vi "Lab2.vi"() -> ()   [LabVIEW 2019]
uses:
  <vilib>/Instr/_visa.llb/VISA Configure Serial Port (Instr).vi
  <vilib>/Utility/file.llb/Write Delimited Spreadsheet (DBL).vi
panel:
  out "Background":bool
  out "Delta":bool
  out "Nominal":bool
  out "UV Index":dbl
  out "array w/ subset deleted":dbl[][](array[numeric])
  out "Lux Index":dbl
  out "UV Chart":dbl(graph)
  out "Lux Chart":dbl(graph)
  in  "?":bool
  in  "Arduino COM Port":refnum<visa-resource-name>="COM3"
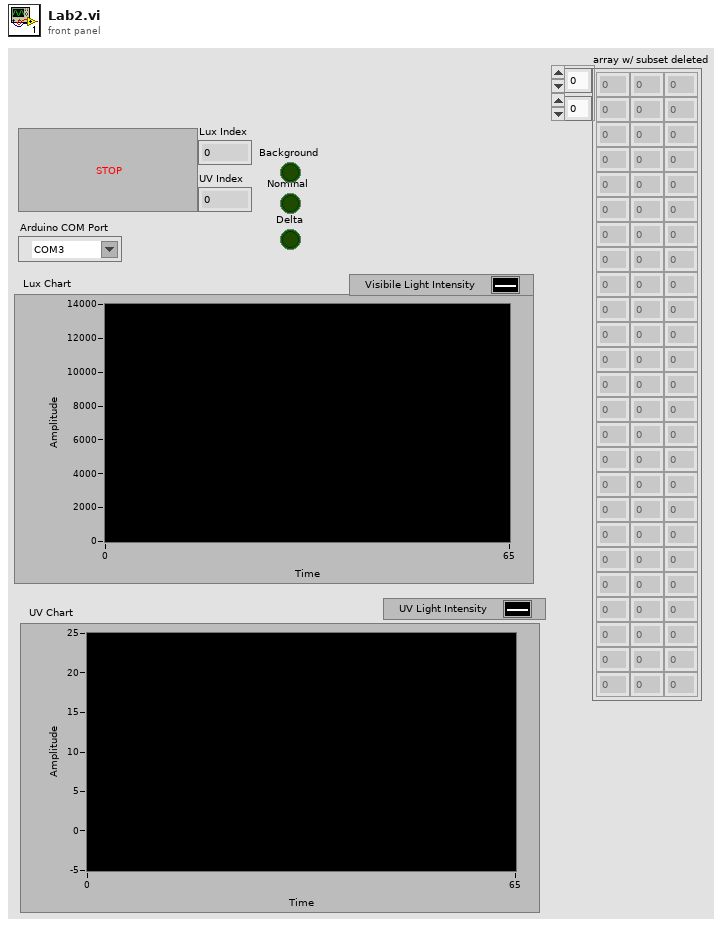
[diagram p1: front panel]
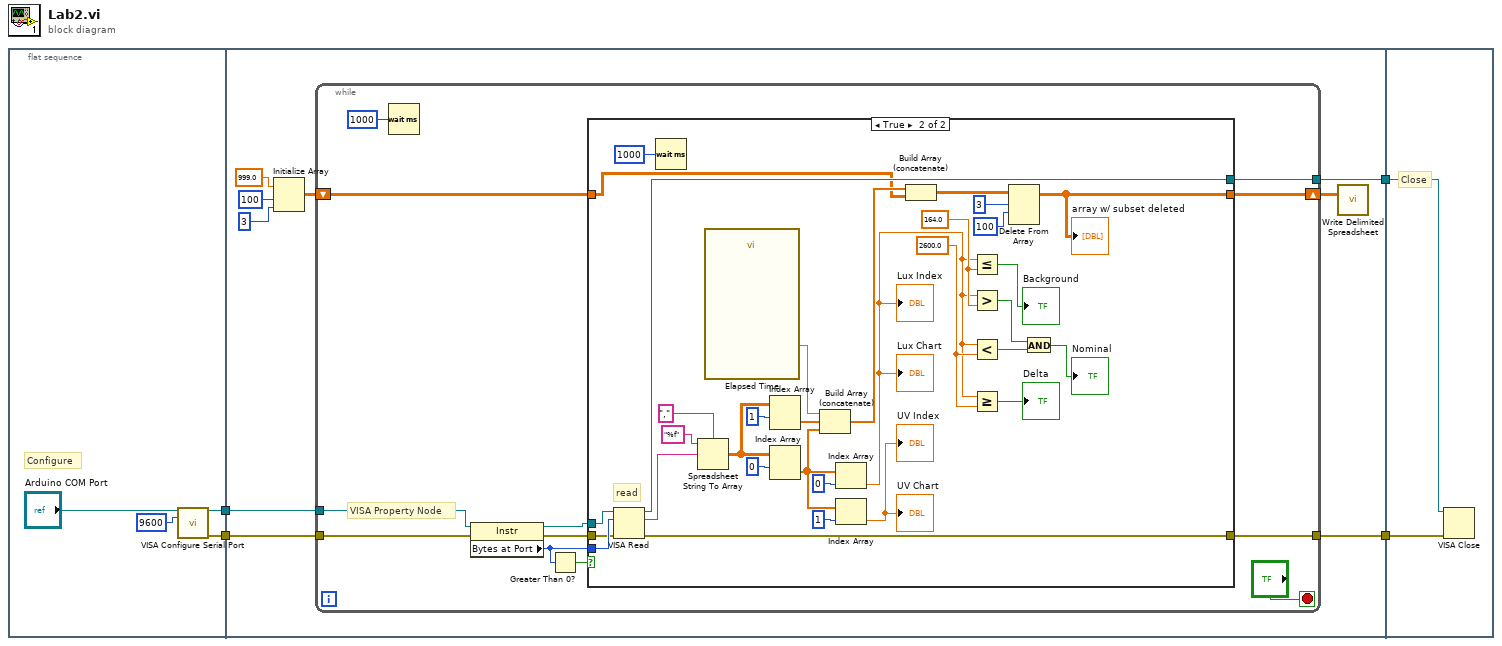
[diagram p0: block diagram]
diagram:
  n1 = flat-sequence {
    tunnel: [w6] -> w4
    tunnel: [w5] -> w3
    tunnel: w4 -> [w17]
    tunnel: [w16] -> w2
    tunnel: w3 -> [w15]
    tunnel: [w14] -> w1
    tunnel: w2 -> [w66]
    tunnel: w1 -> [w65]
    frame #0 {
      # "Configure"
      n2 = call-poly "VISA Configure Serial Port"("VISA resource name"="Arduino COM Port", "baud rate (9600)"=u32 9600) -> ("VISA resource name out"=w6:refnum<visa-resource-name>, "error out"=w5:errorcluster)  [unwired: 12 in]
    }
    frame #1 {
      n3 = Initialize Array(999.0 ("element"), 100 ("dimension size"), 3 ("dimension size")) -> (w10:dbl[][])
      n4 = while {
        tunnel: w17 -> [w21]
        tunnel: [w24] -> w16
        tunnel: w15 -> [w20]
        tunnel: [w22] -> w14
        shift-right: [w18] -> w9
        shift-left: w10 -> [w19]
        stop <- "?" stop-if-true
        # "VISA Property Node"
        n5 = Wait (ms)(milliseconds to wait=u32 1000) -> ()  [unwired: 1 out]
        n6 = property class="Instr"(reference=w21, error in=w20) -> (reference out=w28:refnum<visa-resource-name>, error out=w23:errorcluster, "Bytes at Port"=w27:u32)
        n7 = Greater Than 0?(x=w27) -> (x > 0?=w29:bool)
        n8 = case shown="True" w29 {
          tunnel: w28 -> [w32 w64]
          tunnel: [w32 w63] -> w24
          tunnel: w27 -> [_ w59]
          tunnel: w23 -> [w31 w58]
          tunnel: [w31 w57] -> w22
          tunnel: w19 -> [w30 w50]
          tunnel: [w30 w46] -> w18
          frame False {
          }
          frame True {
            w34 = 2600.0 ("y")
            w39 = 164.0 ("y")
            # "read"
            n9 = VISA Read(VISA resource name=w64, byte count=w59, error in (no error)=w58) -> (VISA resource name out=w63:refnum<visa-resource-name>, read buffer=w62:string, error out=w57:errorcluster)  [unwired: 1 out]
            n10 = Wait (ms)(milliseconds to wait=u32 1000) -> ()  [unwired: 1 out]
            n11 = Spreadsheet String To Array(delimiter (Tab)=",", format string="%f", spreadsheet string=w62) -> (array=w45:dbl[][])  [unwired: 1 in]
            n12 = call "Elapsed Time"() -> ("Elapsed Time (s)"=w53:dbl)  [unwired: 12 in, 7 out]
            n13 = Index Array(array=w45, index (row)=1) -> (element=w52:dbl[])  [unwired: 1 in]
            n14 = Index Array(array=w45, index (row)=0) -> (element=w44:dbl[])  [unwired: 1 in]
            n15 = Build Array (concatenate)(w53, w52, w44) -> (w51:dbl[])
            n16 = Index Array(array=w44, index=0) -> (element=w33:dbl)
            "Lux Chart" <- w33
            "Lux Index" <- w33
            n17 = Index Array(array=w44, index=1) -> (element=→"UV Chart" →"UV Index":dbl)
            n18 = Build Array (concatenate)(w51, w50) -> (w49:dbl[][])
            n19 = Less Or Equal?(x=w33, y=w39) -> (x <= y?=→"Background":bool)
            n20 = Greater?(x=w33, y=w39) -> (0:w38:bool)
            n21 = Less?(x=w33, y=w34) -> (x < y?=w36:bool)
            n22 = Greater Or Equal?(x=w33, y=w34) -> (x >= y?=→"Delta":bool)
            n23 = Delete From Array(array=w49, length=3, index (row)=100) -> (array with subset deleted=w46:dbl[][])  [unwired: 1 in, 1 out]
            "array w/ subset deleted" <- w46
            n24 = And(x=w38, y=w36) -> (x .and. y?=→"Nominal":bool)
          }
        }
      }
      n25 = call-poly <vilib>:"Write Delimited Spreadsheet.vi"("2D data"=w9) -> ()  [unwired: 13 in, 2 out]
    }
    frame #2 {
      # "Close"
      n26 = VISA Close(VISA resource name=w66, error in (no error)=w65) -> ()  [unwired: 1 out]
    }
  }
